vi "Set Word.vi"(0 "OWEN HMI in":refnum<class "OWEN HMI.lvclass">, 5 "address":T1=enum."1 - Level CC", 9 "value":i16, 11 "error in (no error)":errorcluster) -> (4 "OWEN HMI out":refnum<class "OWEN HMI.lvclass">, 15 "error out":errorcluster)   [LabVIEW 2019, in "OWEN HMI.lvclass"]
uses:
  OWEN HMI.lvclass
  Words.ctl
  OWEN HMI.lvclass/OWEN HMI.ctl
  <vilib>/NI/Modbus Library/API/Master/Modbus Master.lvclass
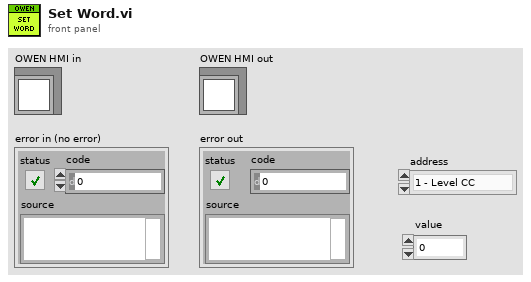
[diagram p1: front panel]
types:
  T1 = typedef "OWEN HMI.lvclass/Words.ctl" = enum16{"0 - Bits", "1 - Level CC", "2 - Temp CC", "3 - Level SO", "4 - Temp SO"}
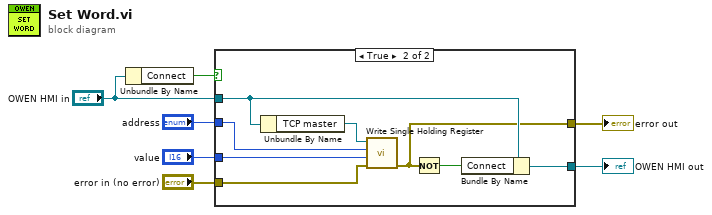
[diagram p0: block diagram]
diagram:
  n1 = Unbundle By Name("OWEN HMI in") -> ("Connect"=w7:bool)
  n2 = case shown="True" w7 {
    tunnel: "error in (no error)" -> [w9 w15]
    tunnel: "OWEN HMI in" -> [w8 w17]
    tunnel: [w8 w12] -> w4
    tunnel: [w9 w11] -> w3
    tunnel: "address" -> [_ w14]
    tunnel: "value" -> [_ w13]
    frame False {
    }
    frame True {
      n3 = Unbundle By Name(w17) -> ("TCP master"=w16:refnum<class "Modbus Master.lvclass">)
      n4 = call-dynamic "Write Single Holding Register.vi"("error in"=w15, "register to write"=w13, "address"=w14, "Modbus master in"=w16) -> ("error out"=w11:errorcluster)  [unwired: 6 in, 1 out]
      n5 = Not(x=w11) -> (.not. x?=w10:bool)
      n6 = Bundle By Name(cluster=w17, "Connect"=w10) -> (w12:refnum<class "OWEN HMI.lvclass">)
    }
  }
  "OWEN HMI out" <- w4
  "error out" <- w3
